vi "exposureTimeSet.vi"(4 "exposureTime (s)":dbl=0.001, 5 "timeDelay(s)":dbl format="%#_6p", 6 "maxExposureTime":dbl=1e-05 caption="Max Exp. Time" format="%#_4ps", 7 "minExposureTime":dbl=1e-05 caption="Min Exp. Time" format="%#_4ps", 8 "exposureUnitsPrefix":dbl=1000000.0 format="%#_6p", 9 "sessionIn":T1) -> (2 "error out":errorcluster, 3 "exposureTimeReadback":dbl)   [LabVIEW 2021]
uses:
  <vilib>/userdefined/High Color/IMAQdx.ctl
  <resource>/objmgr/imaqdx.rc
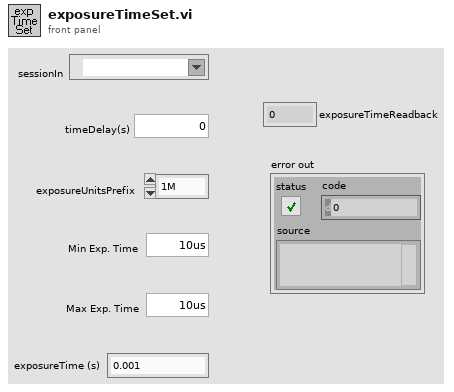
[diagram p1: front panel]
types:
  T1 = typedef "IMAQdx.ctl" = refnum<k21>
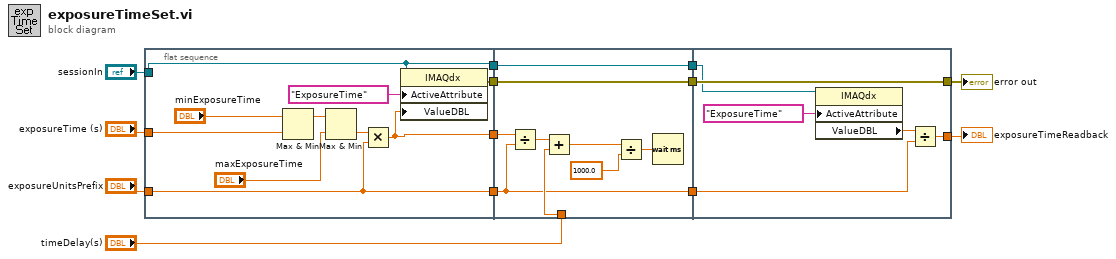
[diagram p0: block diagram]
diagram:
  n1 = flat-sequence {
    tunnel: "exposureTime (s)" -> [w16]
    tunnel: "sessionIn" -> [w14]
    tunnel: [w22] -> w11
    tunnel: "exposureUnitsPrefix" -> [w21]
    tunnel: [w21] -> w9
    tunnel: [w15] -> w5
    tunnel: [w14] -> w1
    tunnel: w11 -> [w30]
    tunnel: w9 -> [w25]
    tunnel: "timeDelay(s)" -> [w27]
    tunnel: [w30] -> w6
    tunnel: w5 -> [w26]
    tunnel: [w25] -> w4
    tunnel: [w24] -> w2
    tunnel: w1 -> [w24]
    tunnel: [w38] -> w8
    tunnel: w6 -> [w38]
    tunnel: w4 -> [w36]
    tunnel: [w35] -> w3
    tunnel: w2 -> [w34]
    frame #0 {
      n2 = Max & Min(x="minExposureTime", y=w16) -> (max(x,y)=w18:dbl)  [unwired: 1 out]
      n3 = Max & Min(x=w18, y="maxExposureTime") -> (min(x,y)=w17:dbl)  [unwired: 1 out]
      n4 = Multiply(x=w17, y=w21) -> (x*y=w15:dbl)
      n5 = property class="IMAQdx"(reference=w14, "ActiveAttribute"="ExposureTime", "ValueDBL"=w15) -> (error out=w22:errorcluster)  [unwired: 1 in, 1 out]
    }
    frame #1 {
      n6 = Divide(x=w26, y=w25) -> (x/y=w28:dbl)
      n7 = Add(x=w28, y=w27) -> (x+y=w29:dbl)
      n8 = Divide(x=w29, y=1000.0) -> (x/y=w32:dbl)
      n9 = Wait (ms)(milliseconds to wait=w32) -> ()  [unwired: 1 out]
    }
    frame #2 {
      n10 = property class="IMAQdx"(reference=w34, "ActiveAttribute"="ExposureTime") -> ("ValueDBL"=w37:dbl)  [unwired: 1 in, 2 out]
      n11 = Divide(x=w37, y=w36) -> (x/y=w35:dbl)
    }
  }
  "exposureTimeReadback" <- w3
  "error out" <- w8
